vi "Write Pane Enable Scrollbars.vi"(10 "Pane":T1, 11 "(FPEN)":refnum<class "(FPEN).lvclass">) -> (3 "(FPEN) Out":refnum<class "(FPEN).lvclass">)   [LabVIEW 2016, in "(FPEN).lvclass"]
uses:
  (FPEN).lvclass
  TypeDefs_Utility/Cluster_FP_Scroll Bars Hide Show.ctl
  TypeDefs_Utility/ENUM_FP_Show-Hide Select.ctl
  (FPEN).lvclass/(FPEN).ctl
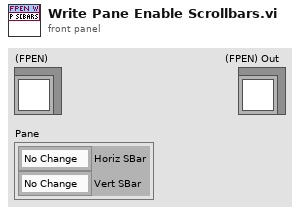
[diagram p1: front panel]
types:
  T1 = typedef "Cluster_FP_Scroll Bars Hide Show.ctl" = cluster{"Horiz SBar":T2, "Vert SBar":T2}
  T2 = typedef "ENUM_FP_Show-Hide Select.ctl" = enum16{"No Change", "Hide", "Show"}
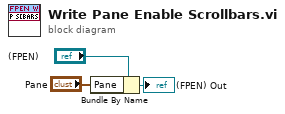
[diagram p0: block diagram]
diagram:
  n1 = Bundle By Name(cluster="(FPEN)", "Pane"="Pane") -> (→"(FPEN) Out":refnum<class "(FPEN).lvclass">)
